vi "Dialog_pw.vi"(11 "String":string) -> (3 "x >= 0?":bool)   [LabVIEW 2022 SP3]
panel:
  out "string":string
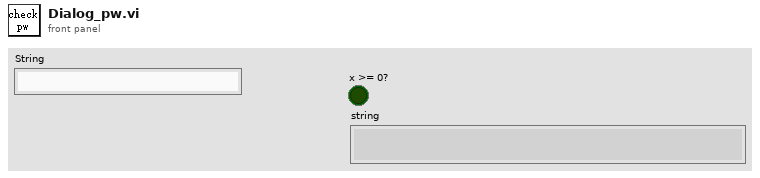
[diagram p1: front panel]
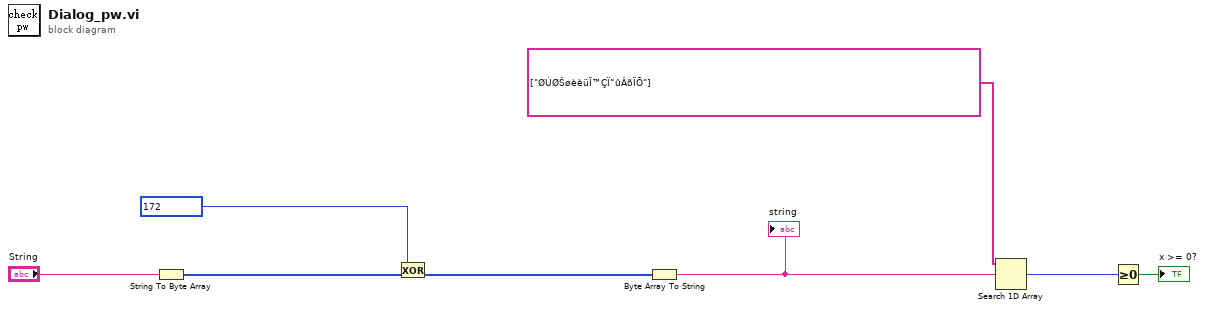
[diagram p0: block diagram]
diagram:
  n1 = String To Byte Array(string="String") -> (unsigned byte array=w7:u8[])
  n2 = Exclusive Or(1:w7, 2:u8 172) -> (0:w5:u8[])
  n3 = Byte Array To String(unsigned byte array=w5) -> (string=w4:string)
  "string" <- w4
  n4 = Search 1D Array(1D array=string[] ["ØÚØŠøèèüÏ™ÇÏ˜ûÂõÏÕ"] ("string"), element=w4) -> (index of element=w2:i32)  [unwired: 1 in]
  n5 = Greater Or Equal To 0?(x=w2) -> (x >= 0?=→"x >= 0?":bool)
